vi "Read SG Pin.vi"(8 "error in (no error)":errorcluster, 11 "ET_Delay_Sweep in":refnum<class "ET_Delay_Sweep.lvclass">) -> (0 "error out":errorcluster, 2 "SG Pin":string, 3 "ET_Delay_Sweep out":refnum<class "ET_Delay_Sweep.lvclass">)   [LabVIEW 2018, in "SeqAuto Evaluations.lvlib" / "ET_Delay_Sweep.lvclass"]
uses:
  ET_Delay_Sweep.lvclass
  ET_Delay_Sweep.lvclass/ET_Delay_Sweep.ctl
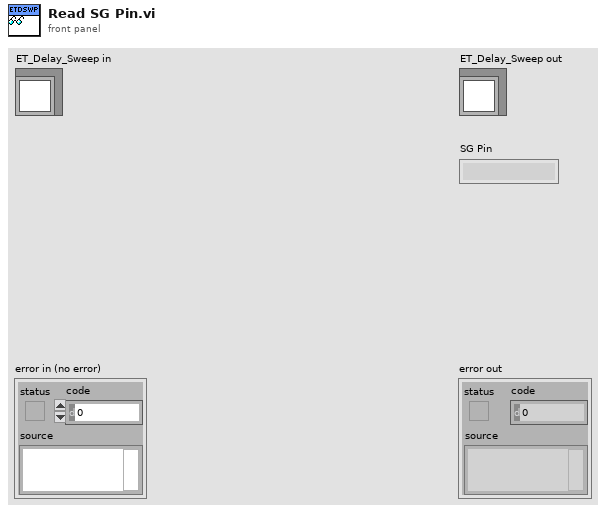
[diagram p1: front panel]
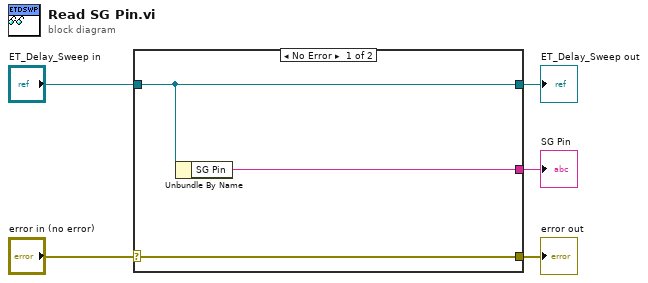
[diagram p0: block diagram]
diagram:
  n1 = case shown="No Error" "error in (no error)" {
    selector: "error in (no error)" -> [w8 w9]
    tunnel: [w8 w9] -> w4
    tunnel: [w7 w10] -> w2
    tunnel: "ET_Delay_Sweep in" -> [w7 w10]
    tunnel: [w6 _] -> w1
    frame No Error {
      n2 = Unbundle By Name(w7) -> ("SG Pin"=w6:string)
    }
    frame Error {
    }
  }
  "error out" <- w4
  "ET_Delay_Sweep out" <- w2
  "SG Pin" <- w1
